vi "Positioncontrol_twomotor_pid.vi"() -> ()   [LabVIEW 2014]
uses:
  <vilib>/rvi/FXPMathLib/FxpSinAndCos/XNode/nifxpmath_SinAndCos.xnode
  <vilib>/eio/EIONode/EIONode.xnode
  <vilib>/rvi/FXPMathLib/FxpMul/XNode/nifxpmath_Multiplier.xnode
  <vilib>/rvi/FXPMathLib/FxpSinAndCos/simVIs/DllFxpSinAndCosTemp_sub.vi
  <vilib>/rvi/FXPMathLib/FxpSinAndCos/subVIs/nifxpmath_SinAndCos_SimConfig.ctl
  <vilib>/rvi/eio/common/nirviEmuTemplateMethod_errors.vi
  <vilib>/rvi/FXPMathLib/sim/FxpSim.dll
  <vilib>/rvi/DataTransferAndStorage/Container/XNode/niFpgaContainer.xnode
  <vilib>/rvi/FXPMathLib/FxpSub/XNode/nifxpmath_Sub.xnode
  <vilib>/rvi/FXPMathLib/FxpAdd/XNode/nifxpmath_Add.xnode
  <vilib>/rvi/Analysis/measure/butterworth/XNode/niFpgaButterworthFilter.xnode
  <vilib>/rvi/interface/RandomDataEmulation/nirviRandomDataFpgaReadWriteTemplate.vi
  <vilib>/rvi/interface/RandomDataEmulation/nirviRandomDataFpgaMultiElementTemplate.vi
panel:
  in  "Ramp_start":bool
  out "Dyr_slope":fxp<+/-,12,8>
  out "Dpr_slope":fxp<+/-,12,8>
  in  "Dyr_end":fxp<+/-,20,10>
  in  "Dyr_time":fxp<+/-,41,11>
  in  "Dpr_end":fxp<+/-,20,10>
  in  "Dpr_time":fxp<+/-,41,11>
  out "Dyr_ramp":fxp<+/-,12,7> format="%.18g"
  out "Dpr_ramp":fxp<+/-,12,7> format="%.18g"
  in  "Dyr_sin/cons":bool
  in  "Dpr_sin/cons":bool
  in  "Sin_magnitude":fxp<+/-,12,8>
  in  "Sin_offset":fxp<+/-,12,8>
  out "Dyr_sin":fxp<+/-,22,7> format="%.18g"
  out "Dpr_sin":fxp<+/-,22,7> format="%.18g"
  in  "Sin_period(sec)":fxp<+,10,8> format="%.21g"
  in  "Time_reset":bool
  in  "coe_ini":bool
  out "Dpt_i":fxp<+/-,25,11>
  out "Dyt_i":fxp<+/-,25,11>
  out "time now":fxp<+/-,41,11>
  in  "D_comp/tune_p":bool
  in  "D_comp/tune_y":bool
  in  "kp t":fxp<+,15,8>
  in  "kp c":fxp<+,15,8>
  in  "Kpp gain":fxp<+,27,10>=0.40625
  in  "Kpp slope gain":fxp<+,20,1>=0.40625
  in  "Kdp 2":fxp<+,27,10>
  in  "Kip 2":fxp<+,27,10>
  in  "I_comp/tune_p":bool
  out "Kpp":fxp<+,12,6>
  out "Kdp":fxp<+,34,10> format="%.25g"
  out "Kip":fxp<+,27,10> format="%.21g"
  in  "tolerance_Dp":fxp<+,12,2>=1.0
  in  "viscous_cons_p":fxp<+/-,20,10>
  in  "fcp":fxp<+/-,15,6>
  in  "fvp":fxp<+,20,12>
  in  "fv_coeff. p":fxp<+,13,1>
  in  "Dp_d_tol":fxp<+,20,12>
  in  "fstp":fxp<+/-,15,6>
  out "Dpr":fxp<+/-,22,7> format="%.18g"
  out "Friction comp_p":fxp<+/-,20,10>
  out "Fp_PID":fxp<+/-,20,10>
  out "Dp_tilde":fxp<+/-,33,9>
  out "xp_d":fxp<+/-,25,15>
  out "Dpt_d":fxp<+/-,25,15>
  out "Dp_d":fxp<+/-,25,15>
  out "vd_p_F":fxp<+/-,20,5>
  out "vq_p_F":fxp<+/-,20,5> format="%.57g"
  in  "Stop motor_p":bool
  out "va_p":fxp<+/-,20,5> format="%.21g"
  out "vb_p":fxp<+/-,20,5> format="%.21g"
  out "omega_p":fxp<+/-,20,9>
  in  "Encoder Reset_p":bool
  out "Encoder Position_p":i32
  out "rad(NrTheta)_p":fxp<+/-,33,18> format="%.21g"
  out "Dp(mm)":fxp<+/-,22,7>
  in  "viscous_cons_y":fxp<+/-,20,10>
  in  "I_comp/tune_y":bool
  in  "fsty":fxp<+/-,15,6>
  out "Dy_d":fxp<+/-,25,15>
  out "Dyr":fxp<+/-,22,7> format="%.18g"
  in  "Dy_d_tol":fxp<+,20,12>
  out "Dy_tilde":fxp<+/-,33,9>
  out "Dyt_d":fxp<+/-,25,15>
  in  "Kiy 2":fxp<+,27,10>
  in  "Kdy 2":fxp<+,27,10>
  in  "ky c":fxp<+,15,8>
  in  "ky t":fxp<+,15,8>
  out "Kiy":fxp<+,27,10> format="%.21g"
  in  "Kpy slope gain":fxp<+,20,1>=0.40625
  in  "Kpy gain":fxp<+,27,10>=0.40625
  in  "fv_coeff. y":fxp<+,13,1>
  out "Friction comp_y":fxp<+/-,20,10>
  in  "fcy":fxp<+/-,15,6>
  in  "fvy":fxp<+,20,12>
  out "xy_d":fxp<+/-,25,15>
  out "AI samp time (us)":u8
  out "x_p":fxp<+/-,30,6> format="%.40g"
  in  "Linear Sensor Reset_y":bool
  in  "kp":fxp<+,15,8>
  out "fp":fxp<+/-,20,10>
  in  "ky":fxp<+,15,8>
  out "fy":fxp<+/-,20,10>
  out "x_y":fxp<+/-,30,6>
  out "Kdy":fxp<+,34,10> format="%.25g"
  out "Kpy":fxp<+,12,6>
  out "Fy_PID":fxp<+/-,20,10>
  in  "tolerance_Dy":fxp<+,12,2>=1.0
  in  "Encoder Reset_y":bool
  out "Encoder Position_y":i32
  out "rad(NrTheta)_y":fxp<+/-,33,18> format="%.21g"
  out "Dy(mm)":fxp<+/-,22,7>
  out "omega_y":fxp<+/-,20,9>
  out "vq_y_F":fxp<+/-,20,5> format="%.57g"
  out "vd_y_F":fxp<+/-,20,5>
  in  "Stop motor_y":bool
  out "va_y":fxp<+/-,20,5> format="%.21g"
  out "vb_y":fxp<+/-,20,5> format="%.21g"
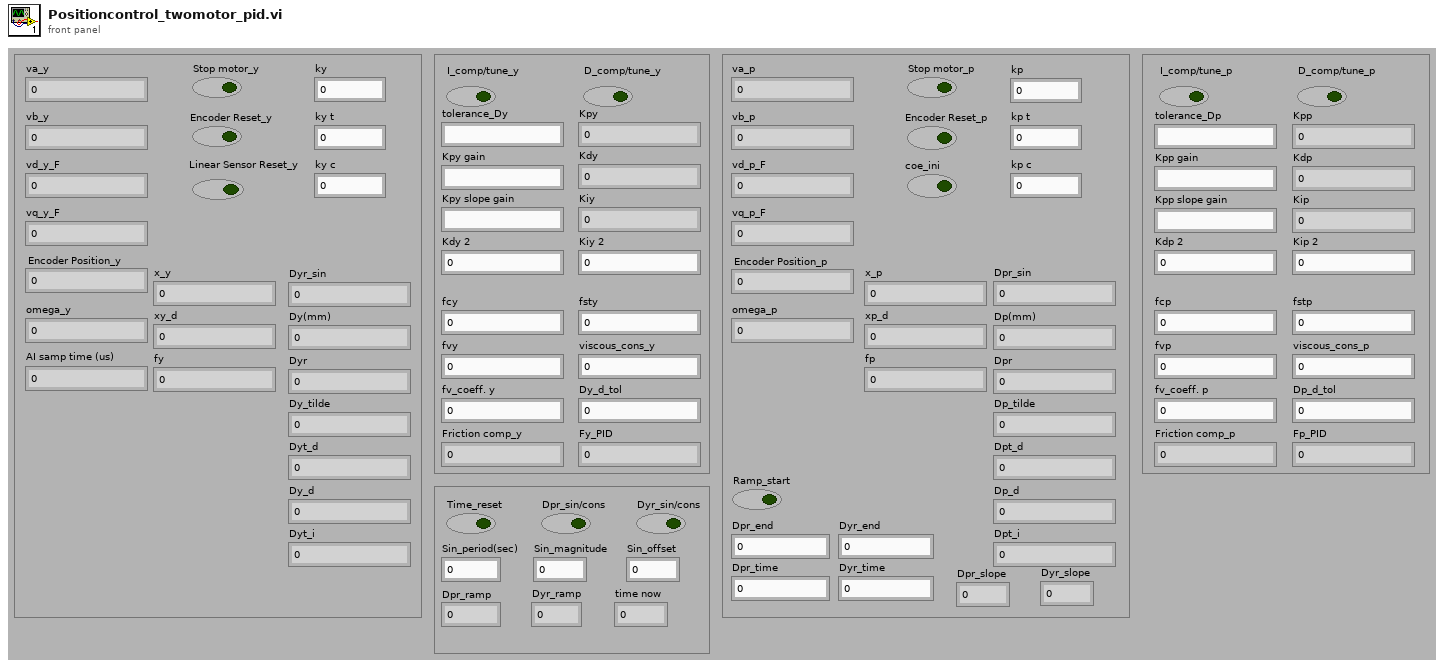
[diagram p1: front panel]
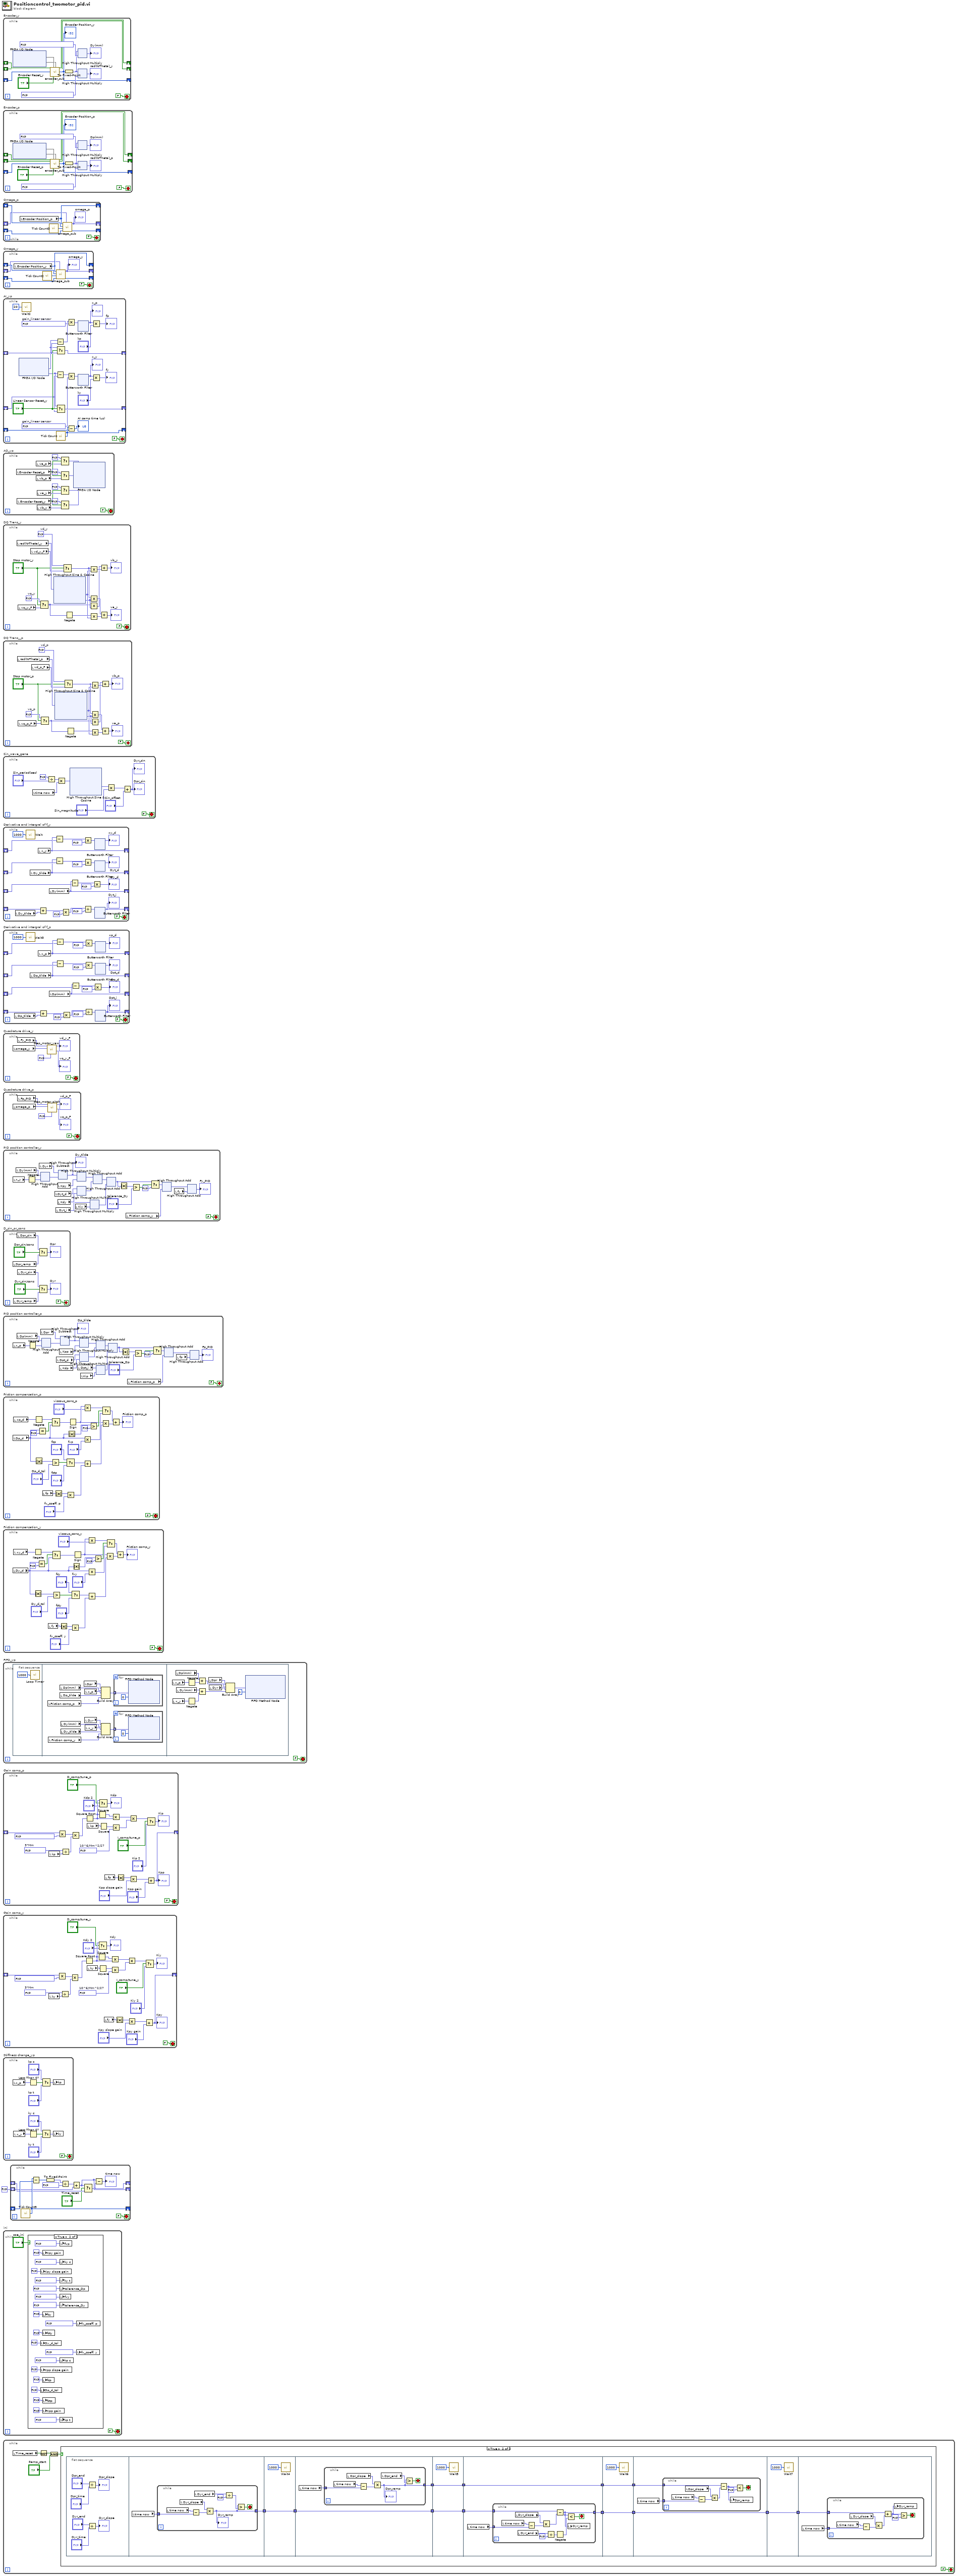
[diagram p0: block diagram]
diagram:
  n1 = while "Encoder_y" {
    shift-right: [w15] -> _
    shift-left: _ -> [w13]
    shift-right: [w14] -> _
    shift-left: _ -> [w12]
    shift-right: [w2] -> _
    shift-left: _ -> [w8]
    stop <- FALSE stop-if-true
    n2 = xnode "FPGA I/O Node"() -> ("Mod3/DIO2"=w11, "Mod3/DIO3"=w10)  [unwired: 2 in, 2 out]
    n3 = call "encoder_sub.vi"("A_pre"=w13, "B_pre"=w12, "Encoder Position_pre"=w8, "A input"=w11, "Encoder Position Reset"="Encoder Reset_y", "B input"=w10) -> ("A"=w15:bool, "B"=w14:bool, "Encoder Position (Counts)"=w2:i32)  [unwired: 19 in]
    "Encoder Position_y" <- w2
    n4 = To Fixed-Point(number=w2) -> (fixed-point=w5:fxp<+/-,18,18>)  [unwired: 1 in]
    n5 = xnode ("High Throughput Multiply")("x"=w5, "y"=fxp<+/-,15,-9> -0.0006049871444702148) -> ("x*y"=→"Dy(mm)":fxp<+/-,21,6>)
    n6 = xnode ("High Throughput Multiply")("x"=w5, "y"=fxp<+,24,0> 0.02499997615814209) -> ("x*y"=→"rad(NrTheta)_y":fxp<+/-,33,18>)
  }
  n7 = while "Encoder_p" {
    shift-right: [w30] -> _
    shift-left: _ -> [w28]
    shift-right: [w29] -> _
    shift-left: _ -> [w27]
    shift-right: [w17] -> _
    shift-left: _ -> [w23]
    stop <- FALSE stop-if-true
    n8 = xnode "FPGA I/O Node"() -> ("Mod3/DIO0"=w26, "Mod3/DIO1"=w25)  [unwired: 2 in, 2 out]
    n9 = call "encoder_sub.vi"("A_pre"=w28, "B_pre"=w27, "Encoder Position_pre"=w23, "A input"=w26, "Encoder Position Reset"="Encoder Reset_p", "B input"=w25) -> ("A"=w30:bool, "B"=w29:bool, "Encoder Position (Counts)"=w17:i32)  [unwired: 19 in]
    "Encoder Position_p" <- w17
    n10 = To Fixed-Point(number=w17) -> (fixed-point=w20:fxp<+/-,18,18>)  [unwired: 1 in]
    n11 = xnode ("High Throughput Multiply")("x"=w20, "y"=fxp<+/-,15,-9> -0.0006049871444702148) -> ("x*y"=→"Dp(mm)":fxp<+/-,21,6>)
    n12 = xnode ("High Throughput Multiply")("x"=w20, "y"=fxp<+,24,0> 0.02499997615814209) -> ("x*y"=→"rad(NrTheta)_p":fxp<+/-,33,18>)
  }
  n13 = while "Omega_p" {
    shift-right: [w39] -> _
    shift-left: _ -> [w38]
    shift-right: [w37] -> _
    shift-left: _ -> [w36]
    shift-right: [w34] -> _
    shift-left: _ -> [w35]
    stop <- FALSE stop-if-true
    n14 = local read "Encoder Position_p"() -> (w39:i32)
    n15 = call "Tick Count3"() -> ("Tick Count(Ticks)"=w32:u32)
    n16 = call "omega_sub.vi"("omega_pre"=w35, "ticks_m_pre"=w36, "ticks"=w32, "count_pre"=w38, "count"=w39) -> ("ticks_m"=w37:u32, "omega"=w34:fxp<+/-,20,9>)  [unwired: 4 in, 1 out]
    "omega_p" <- w34
  }
  n17 = while "Omega_y" {
    shift-right: [w47] -> _
    shift-left: _ -> [w46]
    shift-right: [w45] -> _
    shift-left: _ -> [w44]
    shift-right: [w42] -> _
    shift-left: _ -> [w43]
    stop <- FALSE stop-if-true
    n18 = local read "Encoder Position_y"() -> (w47:i32)
    n19 = call "Tick Count2"() -> ("Tick Count(Ticks)"=w40:u32)
    n20 = call "omega_sub.vi"("omega_pre"=w43, "ticks_m_pre"=w44, "ticks"=w40, "count_pre"=w46, "count"=w47) -> ("ticks_m"=w45:u32, "omega"=w42:fxp<+/-,20,9>)  [unwired: 4 in, 1 out]
    "omega_y" <- w42
  }
  n21 = while "AI_yp" {
    shift-right: [w70] -> _
    shift-left: _ -> [w71]
    shift-right: [w66] -> _
    shift-left: _ -> [w67]
    shift-right: [w61] -> _
    shift-left: _ -> [w60]
    stop <- FALSE stop-if-true
    w48 = fxp<+,25,5> 1.4694995880126953  # gain_linear sensor
    w57 = fxp<+,25,5> 1.5044002532958984  # gain_linear sensor
    n22 = xnode "FPGA I/O Node"() -> ("Mod1/AI0"=w63:fxp<+/-,20,5>, "Mod1/AI1"=w59:fxp<+/-,20,5>)  [unwired: 3 in, 3 out]
    n23 = call "Wait2"("Count(uSec)"=u8 20) -> ()  [unwired: 1 out]
    n24 = Subtract(x=w63, y=w67) -> (x-y=w54:fxp<+/-,21,6>)
    n25 = Subtract(x=w59, y=w60) -> (x-y=w58:fxp<+/-,21,6>)
    n26 = Select(t=w63, s="Linear Sensor Reset_y", f=w67) -> (s? t:f=w66:fxp<+/-,20,5>)
    n27 = Select(t=w59, s="Linear Sensor Reset_y", f=w60) -> (s? t:f=w61:fxp<+/-,20,5>)
    n28 = call "Tick Count"() -> ("Tick Count(uSec)"=w70:u8)
    n29 = Multiply(x=w54, y=w48) -> (x*y=w52:fxp<+/-,30,6>)
    n30 = Multiply(x=w58, y=w57) -> (x*y=w50:fxp<+/-,30,6>)
    n31 = Subtract(x=w70, y=w71) -> (x-y=→"AI samp time (us)":u8)
    n32 = xnode "Butterworth Filter"("input data"=w52) -> ("output data"=w51:fxp<+/-,30,6>)  [unwired: 2 in]
    "x_p" <- w51
    n33 = xnode "Butterworth Filter"("input data"=w50) -> ("output data"=w49:fxp<+/-,30,6>)  [unwired: 2 in]
    "x_y" <- w49
    n34 = Multiply(x=w51, y="kp") -> (x*y=→"fp":fxp<+/-,20,10>)
    n35 = Multiply(x=w49, y="ky") -> (x*y=→"fy":fxp<+/-,20,10>)
  }
  n36 = while "AO_yp" {
    stop <- FALSE stop-if-true
    n37 = local read "Encoder Reset_p"() -> (w101:bool)
    n38 = local read "Encoder Reset_y"() -> (w90:bool)
    n39 = local read "va_p"() -> (w100:fxp<+/-,20,5>)
    n40 = local read "vb_p"() -> (w99:fxp<+/-,20,5>)
    n41 = local read "va_y"() -> (w91:fxp<+/-,20,5>)
    n42 = local read "vb_y"() -> (w92:fxp<+/-,20,5>)
    n43 = Select(t=fxp<+/-,20,5> 5.0 ("Mod2/AO4"), s=w101, f=w100) -> (s? t:f=w96:fxp<+/-,20,5>)
    n44 = Select(t=fxp<+/-,20,5> 0.0 ("Mod2/AO4"), s=w101, f=w99) -> (s? t:f=w95:fxp<+/-,20,5>)
    n45 = Select(t=fxp<+/-,20,5> 5.0 ("Mod2/AO4"), s=w90, f=w91) -> (s? t:f=w89:fxp<+/-,20,5>)
    n46 = Select(t=fxp<+/-,20,5> 0.0 ("Mod2/AO4"), s=w90, f=w92) -> (s? t:f=w88:fxp<+/-,20,5>)
    n47 = xnode "FPGA I/O Node"("Mod2/AO0"=w96, "Mod2/AO1"=w95, "Mod2/AO2"=w89, "Mod2/AO3"=w88) -> ()  [unwired: 4 in, 4 out]
  }
  n48 = while "DQ Trans_y" {
    stop <- FALSE stop-if-true
    w108 = fxp<+/-,20,5> 0.0  # vq_y
    w106 = fxp<+/-,20,5> 0.0  # vd_y
    n49 = local read "rad(NrTheta)_y"() -> (w119:fxp<+/-,33,18>)
    n50 = local read "vq_y_F"() -> (w104:fxp<+/-,20,5>)
    n51 = local read "vd_y_F"() -> (w105:fxp<+/-,20,5>)
    n52 = Select(t=w108, s="Stop motor_y", f=w104) -> (s? t:f=w109:fxp<+/-,20,5>)
    n53 = xnode "High Throughput Sine & Cosine"("x (pi)"=w119) -> ("sin(x)"=w110:fxp<+/-,17,2>, "cos(x)"=w111:fxp<+/-,17,2>)
    n54 = Select(t=w106, s="Stop motor_y", f=w105) -> (s? t:f=w107:fxp<+/-,20,5>)
    n55 = Negate(x=w109) -> (-x=w118:fxp<+/-,21,6>)
    n56 = Multiply(x=w107, y=w110) -> (x*y=w114:fxp<+/-,20,5>)
    n57 = Multiply(x=w107, y=w111) -> (x*y=w117:fxp<+/-,20,5>)
    n58 = Multiply(x=w109, y=w111) -> (x*y=w113:fxp<+/-,20,5>)
    n59 = Multiply(x=w118, y=w110) -> (x*y=w116:fxp<+/-,20,5>)
    n60 = Add(x=w113, y=w114) -> (x+y=→"vb_y":fxp<+/-,20,5>)
    n61 = Add(x=w117, y=w116) -> (x+y=→"va_y":fxp<+/-,20,5>)
  }
  n62 = while "DQ Trans__p" {
    stop <- FALSE stop-if-true
    w158 = fxp<+/-,20,5> 0.0  # vq_p
    w156 = fxp<+/-,20,5> 0.0  # vd_p
    n63 = local read "rad(NrTheta)_p"() -> (w167:fxp<+/-,33,18>)
    n64 = local read "vq_p_F"() -> (w154:fxp<+/-,20,5>)
    n65 = local read "vd_p_F"() -> (w155:fxp<+/-,20,5>)
    n66 = Select(t=w158, s="Stop motor_p", f=w154) -> (s? t:f=w159:fxp<+/-,20,5>)
    n67 = xnode "High Throughput Sine & Cosine"("x (pi)"=w167) -> ("sin(x)"=w160:fxp<+/-,17,2>, "cos(x)"=w161:fxp<+/-,17,2>)
    n68 = Select(t=w156, s="Stop motor_p", f=w155) -> (s? t:f=w157:fxp<+/-,20,5>)
    n69 = Negate(x=w159) -> (-x=w166:fxp<+/-,21,6>)
    n70 = Multiply(x=w157, y=w160) -> (x*y=w163:fxp<+/-,20,5>)
    n71 = Multiply(x=w157, y=w161) -> (x*y=w165:fxp<+/-,20,5>)
    n72 = Multiply(x=w159, y=w161) -> (x*y=w162:fxp<+/-,20,5>)
    n73 = Multiply(x=w166, y=w160) -> (x*y=w164:fxp<+/-,20,5>)
    n74 = Add(x=w162, y=w163) -> (x+y=→"vb_p":fxp<+/-,20,5>)
    n75 = Add(x=w165, y=w164) -> (x+y=→"va_p":fxp<+/-,20,5>)
  }
  n76 = while "Sin_wave_gene" {
    stop <- FALSE stop-if-true
    n77 = local read "time now"() -> (w208:fxp<+/-,41,11>)
    n78 = Divide(x=fxp<+,10,8> 2.0, y="Sin_period(sec)") -> (x/y=w207:fxp<+/-,20,11>)
    n79 = Multiply(x=w207, y=w208) -> (x*y=w206:fxp<+/-,25,11>)
    n80 = xnode "High Throughput Sine & Cosine"("x (pi)"=w206) -> ("sin(x)"=w204:fxp<+/-,17,2>)  [unwired: 1 out]
    n81 = Multiply(x=w204, y="Sin_magnitude") -> (x*y=w202:fxp<+/-,20,8>)
    n82 = Add(x=w202, y="Sin_offset") -> (x+y=→"Dyr_sin" →"Dpr_sin":fxp<+/-,22,7>)
  }
  n83 = while "Derivative and intergral of f_y" {
    shift-right: [w261] -> _
    shift-left: _ -> [w260]
    shift-right: [w257] -> _
    shift-left: _ -> [w258]
    shift-right: [w250] -> _
    shift-left: _ -> [w249]
    shift-right: [w240] -> _
    shift-left: _ -> [w241]
    stop <- FALSE stop-if-true
    n84 = local read "Dy_tilde"() -> (w242:fxp<+/-,33,9>)
    n85 = call "Wait"("Count(uSec)"=u32 1000 ("Count(mSec)")) -> ()  [unwired: 1 out]
    n86 = local read "Dy_tilde"() -> (w257:fxp<+/-,33,9>)
    n87 = local read "x_y"() -> (w261:fxp<+/-,30,6>)
    n88 = Add(x=w241, y=w242) -> (x+y=w243:fxp<+/-,36,12>)
    n89 = local read "Dy(mm)"() -> (w250:fxp<+/-,22,7>)
    n90 = Subtract(x=w261, y=w260) -> (x-y=w263:fxp<+/-,31,7>)
    n91 = Subtract(x=w257, y=w258) -> (x-y=w254:fxp<+/-,34,10>)
    n92 = Multiply(x=w243, y=fxp<+/-,22,12> 0.5) -> (x*y=w245:fxp<+/-,25,15>)
    n93 = Subtract(x=w250, y=w249) -> (x-y=w252:fxp<+/-,23,8>)
    n94 = Multiply(x=w263, y=fxp<+,10,10> 1000.0) -> (x*y=w262:fxp<+/-,25,15>)
    n95 = Multiply(x=w254, y=fxp<+,10,10> 1000.0) -> (x*y=w256:fxp<+/-,25,15>)
    n96 = Divide(x=w245, y=fxp<+/-,25,15> 1000.0) -> (x/y=w247:fxp<+/-,25,11>)
    n97 = Multiply(x=w252, y=fxp<+,10,10> 1000.0) -> (x*y=→"Dy_d":fxp<+/-,25,15>)
    n98 = xnode "Butterworth Filter"("input data"=w262) -> ("output data"=→"xy_d":fxp<+/-,25,15>)  [unwired: 2 in]
    n99 = xnode "Butterworth Filter"("input data"=w256) -> ("output data"=→"Dyt_d":fxp<+/-,25,15>)  [unwired: 2 in]
    n100 = xnode "Butterworth Filter"("input data"=w247) -> ("output data"=w240:fxp<+/-,25,11>)  [unwired: 2 in]
    "Dyt_i" <- w240
  }
  n101 = while "Derivative and intergral of f_p" {
    shift-right: [w312] -> _
    shift-left: _ -> [w311]
    shift-right: [w308] -> _
    shift-left: _ -> [w309]
    shift-right: [w301] -> _
    shift-left: _ -> [w300]
    shift-right: [w291] -> _
    shift-left: _ -> [w292]
    stop <- FALSE stop-if-true
    n102 = local read "Dp_tilde"() -> (w298:fxp<+/-,33,9>)
    n103 = call "Wait3"("Count(uSec)"=u32 1000 ("Count(mSec)")) -> ()  [unwired: 1 out]
    n104 = local read "Dp_tilde"() -> (w308:fxp<+/-,33,9>)
    n105 = local read "x_p"() -> (w312:fxp<+/-,30,6>)
    n106 = Add(x=w292, y=w298) -> (x+y=w297:fxp<+/-,36,12>)
    n107 = local read "Dp(mm)"() -> (w301:fxp<+/-,22,7>)
    n108 = Subtract(x=w312, y=w311) -> (x-y=w314:fxp<+/-,31,7>)
    n109 = Subtract(x=w308, y=w309) -> (x-y=w305:fxp<+/-,34,10>)
    n110 = Multiply(x=w297, y=fxp<+/-,22,12> 0.5) -> (x*y=w295:fxp<+/-,25,15>)
    n111 = Subtract(x=w301, y=w300) -> (x-y=w303:fxp<+/-,23,8>)
    n112 = Multiply(x=w314, y=fxp<+,10,10> 1000.0) -> (x*y=w313:fxp<+/-,25,15>)
    n113 = Multiply(x=w305, y=fxp<+,10,10> 1000.0) -> (x*y=w307:fxp<+/-,25,15>)
    n114 = Divide(x=w295, y=fxp<+/-,25,15> 1000.0) -> (x/y=w293:fxp<+/-,25,11>)
    n115 = Multiply(x=w303, y=fxp<+,10,10> 1000.0) -> (x*y=→"Dp_d":fxp<+/-,25,15>)
    n116 = xnode "Butterworth Filter"("input data"=w313) -> ("output data"=→"xp_d":fxp<+/-,25,15>)  [unwired: 2 in]
    n117 = xnode "Butterworth Filter"("input data"=w307) -> ("output data"=→"Dpt_d":fxp<+/-,25,15>)  [unwired: 2 in]
    n118 = xnode "Butterworth Filter"("input data"=w293) -> ("output data"=w291:fxp<+/-,25,11>)  [unwired: 2 in]
    "Dpt_i" <- w291
  }
  n119 = while "Quadrature drive_y" {
    stop <- FALSE stop-if-true
    n120 = local read "omega_y"() -> (w345:fxp<+/-,20,9>)
    n121 = local read "Fy_PID"() -> (w346:fxp<+/-,20,10>)
    n122 = call "step_motor_yaw.vi"("F_Threshold"=fxp<+,12,12> 10.0, "omega_y"=w345, "F"=w346) -> ("vq_F"=→"vq_y_F":fxp<+/-,20,5>, "vd_F"=→"vd_y_F":fxp<+/-,20,5>)  [unwired: 7 in]
  }
  n123 = while "Quadrature drive_p" {
    stop <- FALSE stop-if-true
    n124 = local read "omega_p"() -> (w350:fxp<+/-,20,9>)
    n125 = local read "Fp_PID"() -> (w352:fxp<+/-,20,10>)
    n126 = call "step_motor_pitch.vi"("F_Threshold"=fxp<+,12,12> 10.0, "omega_p"=w350, "F"=w352) -> ("vq_F"=→"vq_p_F":fxp<+/-,20,5>, "vd_F"=→"vd_p_F":fxp<+/-,20,5>)  [unwired: 7 in]
  }
  n127 = while "PID position controller_y" {
    stop <- FALSE stop-if-true
    n128 = local read "x_y"() -> (w356:fxp<+/-,30,6>)
    n129 = local read "Dy(mm)"() -> (w355:fxp<+/-,22,7>)
    n130 = Negate(x=w356) -> (-x=w357:fxp<+/-,31,7>)
    n131 = local read "Dyr"() -> (w370:fxp<+/-,22,7>)
    n132 = xnode ("High Throughput Add")("x"=w355, "y"=w357) -> ("x+y"=w354:fxp<+/-,32,8>)
    n133 = local read "Dyt_d"() -> (w366:fxp<+/-,25,15>)
    n134 = local read "Dyt_i"() -> (w364:fxp<+/-,25,11>)
    n135 = local read "Kpy"() -> (w368:fxp<+,12,6>)
    n136 = local read "Kdy"() -> (w367:fxp<+,34,10>)
    n137 = xnode "High Throughput Subtract"("x"=w370, "y"=w354) -> ("x-y"=w369:fxp<+/-,33,9>)
    "Dy_tilde" <- w369
    n138 = local read "Kiy"() -> (w365:fxp<+,27,10>)
    n139 = xnode ("High Throughput Multiply")("x"=w369, "y"=w368) -> ("x*y"=w363:fxp<+/-,45,15>)
    n140 = xnode ("High Throughput Multiply")("x"=w366, "y"=w367) -> ("x*y"=w362:fxp<+/-,59,25>)
    n141 = xnode ("High Throughput Multiply")("x"=w364, "y"=w365) -> ("x*y"=w361:fxp<+/-,52,21>)
    n142 = xnode ("High Throughput Add")("x"=w363, "y"=w362) -> ("x+y"=w360:fxp<+/-,60,26>)
    n143 = xnode ("High Throughput Add")("x"=w360, "y"=w361) -> ("x+y"=w359:fxp<+/-,20,10>)
    n144 = Absolute Value(x=w359) -> (abs(x)=w377:fxp<+,20,10>)
    n145 = local read "Friction comp_y"() -> (w371:fxp<+/-,20,10>)
    n146 = Greater?(x=w377, y="tolerance_Dy") -> (0:w376:bool)
    n147 = Select(t=w359, s=w376, f=fxp<+/-,20,10> 0.0) -> (s? t:f=w373:fxp<+/-,20,10>)
    n148 = xnode ("High Throughput Add")("x"=w373, "y"=w371) -> ("x+y"=w372:fxp<+/-,20,10>)
    n149 = local read "fy"() -> (w374:fxp<+/-,20,10>)
    n150 = xnode ("High Throughput Add")("x"=w372, "y"=w374) -> ("x+y"=→"Fy_PID":fxp<+/-,20,10>)
  }
  n151 = while "D_sin_or_cons" {
    stop <- FALSE stop-if-true
    n152 = local read "Dpr_ramp"() -> (w381:fxp<+/-,12,7>)
    n153 = local read "Dyr_ramp"() -> (w380:fxp<+/-,12,7>)
    n154 = local read "Dpr_sin"() -> (w383:fxp<+/-,22,7>)
    n155 = local read "Dyr_sin"() -> (w382:fxp<+/-,22,7>)
    n156 = Select(t=w383, s="Dpr_sin/cons", f=w381) -> (s? t:f=→"Dpr":fxp<+/-,22,7>)
    n157 = Select(t=w382, s="Dyr_sin/cons", f=w380) -> (s? t:f=→"Dyr":fxp<+/-,22,7>)
  }
  n158 = while "PID position controller_p" {
    stop <- FALSE stop-if-true
    n159 = local read "x_p"() -> (w392:fxp<+/-,30,6>)
    n160 = local read "Dp(mm)"() -> (w390:fxp<+/-,22,7>)
    n161 = Negate(x=w392) -> (-x=w391:fxp<+/-,31,7>)
    n162 = local read "Dpr"() -> (w403:fxp<+/-,22,7>)
    n163 = xnode ("High Throughput Add")("x"=w390, "y"=w391) -> ("x+y"=w389:fxp<+/-,32,8>)
    n164 = local read "Dpt_d"() -> (w406:fxp<+/-,25,15>)
    n165 = local read "Kpp"() -> (w404:fxp<+,12,6>)
    n166 = local read "Kdp"() -> (w405:fxp<+,34,10>)
    n167 = xnode "High Throughput Subtract"("x"=w403, "y"=w389) -> ("x-y"=w399:fxp<+/-,33,9>)
    "Dp_tilde" <- w399
    n168 = local read "Dpt_i"() -> (w408:fxp<+/-,25,11>)
    n169 = xnode ("High Throughput Multiply")("x"=w399, "y"=w404) -> ("x*y"=w409:fxp<+/-,45,15>)
    n170 = xnode ("High Throughput Multiply")("x"=w406, "y"=w405) -> ("x*y"=w410:fxp<+/-,59,25>)
    n171 = local read "Kip"() -> (w407:fxp<+,27,10>)
    n172 = xnode ("High Throughput Add")("x"=w409, "y"=w410) -> ("x+y"=w412:fxp<+/-,60,26>)
    n173 = xnode ("High Throughput Multiply")("x"=w408, "y"=w407) -> ("x*y"=w411:fxp<+/-,52,21>)
    n174 = xnode ("High Throughput Add")("x"=w412, "y"=w411) -> ("x+y"=w413:fxp<+/-,20,10>)
    n175 = Absolute Value(x=w413) -> (abs(x)=w400:fxp<+,20,10>)
    n176 = local read "Friction comp_p"() -> (w396:fxp<+/-,20,10>)
    n177 = Greater?(x=w400, y="tolerance_Dp") -> (0:w401:bool)
    n178 = Select(t=w413, s=w401, f=fxp<+/-,20,10> 0.0) -> (s? t:f=w397:fxp<+/-,20,10>)
    n179 = xnode ("High Throughput Add")("x"=w397, "y"=w396) -> ("x+y"=w394:fxp<+/-,20,10>)
    n180 = local read "fp"() -> (w395:fxp<+/-,20,10>)
    n181 = xnode ("High Throughput Add")("x"=w394, "y"=w395) -> ("x+y"=→"Fp_PID":fxp<+/-,20,10>)
  }
  n182 = while "Friction compensation_p" {
    stop <- FALSE stop-if-true
    n183 = local read "Dp_d"() -> (w421:fxp<+/-,25,15>)
    n184 = local read "xp_d"() -> (w416:fxp<+/-,25,15>)
    n185 = Negate(x=w416) -> (-x=w415:fxp<+/-,26,16>)
    n186 = Absolute Value(x=w421) -> (abs(x)=w434:fxp<+,25,15>)
    n187 = Equal?(x=w421, y=fxp<+/-,25,15> 0.0) -> (x = y?=w422:bool)
    n188 = local read "fp"() -> (w439:fxp<+/-,20,10>)
    n189 = Greater?(x=w434, y="Dp_d_tol") -> (0:w433:bool)
    n190 = Select(t=w415, s=w422, f=w421) -> (s? t:f=w420:fxp<+/-,26,16>)
    n191 = Absolute Value(x=w439) -> (abs(x)=w440:fxp<+,20,10>)
    n192 = Select(t="fcp", s=w433, f="fstp") -> (s? t:f=w431:fxp<+/-,15,6>)
    n193 = Multiply(x=w440, y="fv_coeff. p") -> (x*y=w438:fxp<+/-,20,10>)
    n194 = Absolute Value(x=w421) -> (abs(x)=w428:fxp<+,25,15>)
    n195 = Sign(1:w420) -> (0:w419:fxp<+/-,2,2>)
    n196 = Multiply(x=w419, y="viscous_cons_p") -> (x*y=w424:fxp<+/-,20,10>)
    n197 = Multiply(x=w421, y="fvp") -> (x*y=w426:fxp<+/-,20,10>)
    n198 = Add(x=w431, y=w438) -> (x+y=w437:fxp<+/-,20,10>)
    n199 = Greater?(x=w428, y=fxp<+/-,25,15> 25.0) -> (0:w427:bool)
    n200 = Multiply(x=w419, y=w437) -> (x*y=w436:fxp<+/-,20,10>)
    n201 = Select(t=w424, s=w427, f=w426) -> (s? t:f=w425:fxp<+/-,20,10>)
    n202 = Add(x=w425, y=w436) -> (x+y=→"Friction comp_p":fxp<+/-,20,10>)
  }
  n203 = while "Friction compensation_y" {
    stop <- FALSE stop-if-true
    n204 = local read "Dy_d"() -> (w448:fxp<+/-,25,15>)
    n205 = local read "xy_d"() -> (w445:fxp<+/-,25,15>)
    n206 = Negate(x=w445) -> (-x=w444:fxp<+/-,26,16>)
    n207 = Absolute Value(x=w448) -> (abs(x)=w462:fxp<+,25,15>)
    n208 = Equal?(x=w448, y=fxp<+/-,25,15> 0.0) -> (x = y?=w449:bool)
    n209 = local read "fy"() -> (w468:fxp<+/-,20,10>)
    n210 = Select(t=w444, s=w449, f=w448) -> (s? t:f=w447:fxp<+/-,26,16>)
    n211 = Greater?(x=w462, y="Dy_d_tol") -> (0:w461:bool)
    n212 = Absolute Value(x=w468) -> (abs(x)=w469:fxp<+,20,10>)
    n213 = Multiply(x=w469, y="fv_coeff. y") -> (x*y=w466:fxp<+/-,20,10>)
    n214 = Select(t="fcy", s=w461, f="fsty") -> (s? t:f=w459:fxp<+/-,15,6>)
    n215 = Absolute Value(x=w448) -> (abs(x)=w456:fxp<+,25,15>)
    n216 = Sign(1:w447) -> (0:w446:fxp<+/-,2,2>)
    n217 = Multiply(x=w446, y="viscous_cons_y") -> (x*y=w451:fxp<+/-,20,10>)
    n218 = Multiply(x=w448, y="fvy") -> (x*y=w454:fxp<+/-,20,10>)
    n219 = Add(x=w459, y=w466) -> (x+y=w465:fxp<+/-,20,10>)
    n220 = Greater?(x=w456, y=fxp<+/-,25,15> 25.0) -> (0:w455:bool)
    n221 = Multiply(x=w446, y=w465) -> (x*y=w464:fxp<+/-,20,10>)
    n222 = Select(t=w451, s=w455, f=w454) -> (s? t:f=w453:fxp<+/-,20,10>)
    n223 = Add(x=w453, y=w464) -> (x+y=→"Friction comp_y":fxp<+/-,20,10>)
  }
  n224 = while "FIFO_yp" {
    stop <- FALSE stop-if-true
    n225 = flat-sequence {
      frame #0 {
        n226 = call "Loop Timer"("Count(uSec)"=u32 1000 ("Loop Period (usec)")) -> ()  [unwired: 1 out]
      }
      frame #1 {
        n227 = local read "Friction comp_p"() -> (w476:fxp<+/-,20,10>)
        n228 = local read "Friction comp_y"() -> (w485:fxp<+/-,20,10>)
        n229 = local read "Dp(mm)"() -> (w479:fxp<+/-,22,7>)
        n230 = local read "Dp_tilde"() -> (w477:fxp<+/-,33,9>)
        n231 = local read "Dy(mm)"() -> (w482:fxp<+/-,22,7>)
        n232 = local read "Dy_tilde"() -> (w484:fxp<+/-,33,9>)
        n233 = local read "Dpr"() -> (w480:fxp<+/-,22,7>)
        n234 = local read "x_p"() -> (w478:fxp<+/-,30,6>)
        n235 = local read "Dyr"() -> (w481:fxp<+/-,22,7>)
        n236 = local read "x_y"() -> (w483:fxp<+/-,30,6>)
        n237 = Build Array(w480, w479, w478, w477, w476) -> (w475:fxp<+/-,34,10>[])
        n238 = Build Array(w481, w482, w483, w484, w485) -> (w486:fxp<+/-,34,10>[])
        n239 = for {
          tunnel: w475 -> [w487] mode=indexing
          n240 = xnode ("FIFO Method Node")("Element"=w487, "Timeout"=0) -> ()  [unwired: 1 in, 2 out]
        }
        n241 = for {
          tunnel: w486 -> [w489] mode=indexing
          n242 = xnode ("FIFO Method Node")("Element"=w489, "Timeout"=0) -> ()  [unwired: 1 in, 2 out]
        }
      }
      frame #2 {
        n243 = local read "x_p"() -> (w502:fxp<+/-,30,6>)
        n244 = local read "x_y"() -> (w493:fxp<+/-,30,6>)
        n245 = local read "Dp(mm)"() -> (w500:fxp<+/-,22,7>)
        n246 = local read "Dy(mm)"() -> (w495:fxp<+/-,22,7>)
        n247 = Negate(x=w502) -> (-x=w501:fxp<+/-,31,7>)
        n248 = Negate(x=w493) -> (-x=w494:fxp<+/-,31,7>)
        n249 = Add(x=w500, y=w501) -> (x+y=w498:fxp<+/-,32,8>)
        n250 = Add(x=w495, y=w494) -> (x+y=w492:fxp<+/-,32,8>)
        n251 = local read "Dpr"() -> (w499:fxp<+/-,22,7>)
        n252 = local read "Dyr"() -> (w491:fxp<+/-,22,7>)
        n253 = Build Array(w499, w498, w491, w492) -> (w497:fxp<+/-,32,8>[])
        n254 = xnode ("FIFO Method Node")("Element"=w497, "Timeout"=0) -> ()  [unwired: 1 in, 2 out]
      }
    }
  }
  n255 = while "Gain comp_p" {
    shift-right: [w507] -> _
    shift-left: _ -> [w526]
    stop <- FALSE stop-if-true
    w514 = fxp<+,14,7> 111.8125  # 10^6/Mm^2/27
    w529 = fxp<+,14,7> 54.6015625  # 3*Mm
    n256 = local read "kp"() -> (w528:fxp<+,15,8>)
    n257 = Multiply(x=w526, y=fxp<+,12,-6> 0.00099945068359375) -> (x*y=w525:fxp<+,24,0>)
    n258 = Divide(x=w529, y=w528) -> (x/y=w524:fxp<+,23,7>)
    n259 = Multiply(x=w525, y=w524) -> (x*y=w523:fxp<+,32,0>)
    n260 = Square Root(x=w523) -> (sqrt(x)=w510:fxp<+,26,2>)
    n261 = local read "kp"() -> (w515:fxp<+,15,8>)
    n262 = Square(x=w510) -> (x^2=w517:fxp<+,27,3>)
    n263 = Select(t=w510, s="D_comp/tune_p", f="Kdp 2") -> (s? t:f=→"Kdp":fxp<+,34,10>)
    n264 = Square(x=w515) -> (x^2=w513:fxp<+,30,16>)
    n265 = local read "fp"() -> (w520:fxp<+/-,20,10>)
    n266 = Multiply(x=w517, y=w510) -> (x*y=w516:fxp<+,27,3>)
    n267 = Multiply(x=w513, y=w514) -> (x*y=w512:fxp<+,44,20>)
    n268 = Absolute Value(x=w520) -> (abs(x)=w521:fxp<+,20,10>)
    n269 = Multiply(x=w516, y=w512) -> (x*y=w509:fxp<+,27,10>)
    n270 = Multiply(x=w521, y="Kpp slope gain") -> (x*y=w519:fxp<+,12,4>)
    n271 = Add(x=w519, y="Kpp gain") -> (x+y=w507:fxp<+,12,6>)
    "Kpp" <- w507
    n272 = Select(t=w509, s="I_comp/tune_p", f="Kip 2") -> (s? t:f=→"Kip":fxp<+,27,10>)
  }
  n273 = while "Gain comp_y" {
    shift-right: [w545] -> _
    shift-left: _ -> [w554]
    stop <- FALSE stop-if-true
    w541 = fxp<+,14,7> 111.8125  # 10^6/Mm^2/27
    w557 = fxp<+,14,7> 54.6015625  # 3*Mm
    n274 = local read "ky"() -> (w556:fxp<+,15,8>)
    n275 = Multiply(x=w554, y=fxp<+,12,-6> 0.00099945068359375) -> (x*y=w553:fxp<+,24,0>)
    n276 = Divide(x=w557, y=w556) -> (x/y=w552:fxp<+,23,7>)
    n277 = Multiply(x=w553, y=w552) -> (x*y=w551:fxp<+,32,0>)
    n278 = Square Root(x=w551) -> (sqrt(x)=w536:fxp<+,26,2>)
    n279 = local read "ky"() -> (w542:fxp<+,15,8>)
    n280 = Square(x=w536) -> (x^2=w544:fxp<+,27,3>)
    n281 = Select(t=w536, s="D_comp/tune_y", f="Kdy 2") -> (s? t:f=→"Kdy":fxp<+,34,10>)
    n282 = Square(x=w542) -> (x^2=w540:fxp<+,30,16>)
    n283 = local read "fy"() -> (w548:fxp<+/-,20,10>)
    n284 = Multiply(x=w544, y=w536) -> (x*y=w543:fxp<+,27,3>)
    n285 = Multiply(x=w540, y=w541) -> (x*y=w539:fxp<+,44,20>)
    n286 = Absolute Value(x=w548) -> (abs(x)=w549:fxp<+,20,10>)
    n287 = Multiply(x=w543, y=w539) -> (x*y=w534:fxp<+,27,10>)
    n288 = Multiply(x=w549, y="Kpy slope gain") -> (x*y=w547:fxp<+,12,4>)
    n289 = Add(x=w547, y="Kpy gain") -> (x+y=w545:fxp<+,12,6>)
    "Kpy" <- w545
    n290 = Select(t=w534, s="I_comp/tune_y", f="Kiy 2") -> (s? t:f=→"Kiy":fxp<+,27,10>)
  }
  n291 = while "Stiffness change_yp" {
    stop <- FALSE stop-if-true
    n292 = local read "x_p"() -> (w559:fxp<+/-,30,6>)
    n293 = local read "x_y"() -> (w569:fxp<+/-,30,6>)
    n294 = Less Than 0?(x=w559) -> (x < 0?=w560:bool)
    n295 = Less Than 0?(x=w569) -> (x < 0?=w568:bool)
    n296 = Select(t="kp c", s=w560, f="kp t") -> (s? t:f=w561:fxp<+,15,8>)
    n297 = Select(t="ky c", s=w568, f="ky t") -> (s? t:f=w567:fxp<+,15,8>)
    n298 = local write "kp"(w561) -> ()
    n299 = local write "ky"(w567) -> ()
  }
  n300 = while "ini" {
    stop <- FALSE stop-if-true
    n301 = case shown="True" "coe_ini" {
      frame False {
      }
      frame True {
        n302 = local write "Kpy slope gain"(fxp<+,20,1> 0.0 ("Kpy slope gain")) -> ()
        n303 = local write "Dy_d_tol"(fxp<+,20,12> 3.0 ("Dy_d_tol")) -> ()
        n304 = local write "Kpp slope gain"(fxp<+,20,1> 0.0 ("Kpp slope gain")) -> ()
        n305 = local write "Dp_d_tol"(fxp<+,20,12> 3.0 ("Dp_d_tol")) -> ()
        n306 = local write "Kpy gain"(fxp<+,27,10> 10.0 ("Kpy gain")) -> ()
        n307 = local write "fcy"(fxp<+/-,15,6> 18.0 ("fcy")) -> ()
        n308 = local write "fsty"(fxp<+/-,15,6> 18.0 ("fsty")) -> ()
        n309 = local write "fcp"(fxp<+/-,15,6> 14.0 ("fcp")) -> ()
        n310 = local write "fstp"(fxp<+/-,15,6> 16.0 ("fstp")) -> ()
        n311 = local write "Kpp gain"(fxp<+,27,10> 10.0 ("Kpp gain")) -> ()
        n312 = local write "fvp"(fxp<+,20,12> 0.19921875 ("fvp")) -> ()
        n313 = local write "ky c"(fxp<+,15,8> 34.0234375 ("kp c")) -> ()
        n314 = local write "ky t"(fxp<+,15,8> 33.3359375 ("ky")) -> ()
        n315 = local write "tolerance_Dp"(fxp<+,12,2> 0.099609375 ("tolerance_p")) -> ()
        n316 = local write "fvy"(fxp<+,20,12> 0.19921875 ("fvy")) -> ()
        n317 = local write "tolerance_Dy"(fxp<+,12,2> 0.099609375 ("tolerance_y")) -> ()
        n318 = local write "kp c"(fxp<+,15,8> 36.2421875 ("kp c")) -> ()
        n319 = local write "kp t"(fxp<+,15,8> 31.8046875 ("kp t")) -> ()
        n320 = local write "fv_coeff. p"(fxp<+,13,1> 0.14990234375 ("fv_coeff. p")) -> ()
        n321 = local write "fv_coeff. y"(fxp<+,13,1> 0.14990234375 ("fv_coeff. y")) -> ()
      }
    }
  }
  n322 = while {
    stop <- FALSE stop-if-true
    n323 = local read "Time_reset"() -> (w595:bool)
    n324 = Not(x=w595) -> (.not. x?=w593:bool)
    n325 = And(x=w593, y="Ramp_start") -> (x .and. y?=w592:bool)
    n326 = case shown="True" w592 {
      frame False {
      }
      frame True {
        n327 = flat-sequence {
          tunnel: [w616] -> w608
          tunnel: w608 -> [w626]
          tunnel: [w626] -> w607
          tunnel: [w630] -> w606
          tunnel: w607 -> [w630]
          tunnel: [w629] -> w605
          tunnel: [w639] -> w604
          tunnel: w606 -> [w639]
          tunnel: [w638] -> w603
          tunnel: w605 -> [w638]
          tunnel: w604 -> [w644]
          tunnel: [w643] -> w602
          tunnel: w603 -> [w643]
          tunnel: [w642] -> w601
          tunnel: [w658] -> w600
          tunnel: w602 -> [w658]
          tunnel: w601 -> [w657]
          tunnel: [w657] -> w599
          tunnel: w600 -> [w662]
          tunnel: w599 -> [w661]
          tunnel: [w661] -> w598
          tunnel: w598 -> [w673]
          tunnel: [w673] -> w597
          tunnel: w597 -> [w675]
          frame #0 {
            n328 = Divide(x="Dpr_end", y="Dpr_time") -> (x/y=→"Dpr_slope":fxp<+/-,12,8>)
            n329 = Divide(x="Dyr_end", y="Dyr_time") -> (x/y=→"Dyr_slope":fxp<+/-,12,8>)
          }
          frame #1 {
            n330 = local read "time now"() -> (w615:fxp<+/-,41,11>)
            n331 = while {
              tunnel: [w621] -> w616
              tunnel: w615 -> [w618]
              stop <- w622 stop-if-true
              n332 = local read "time now"() -> (w619:fxp<+/-,41,11>)
              n333 = local read "Dyr_slope"() -> (w620:fxp<+/-,12,8>)
              n334 = Subtract(x=w619, y=w618) -> (x-y=w617:fxp<+/-,42,12>)
              n335 = local read "Dyr_end"() -> (w625:fxp<+/-,20,10>)
              n336 = Multiply(x=w620, y=w617) -> (x*y=w621:fxp<+/-,12,7>)
              "Dyr_ramp" <- w621
              n337 = Divide(x=w625, y=fxp<+/-,20,10> 2.0) -> (x/y=w623:fxp<+/-,41,21>)
              n338 = Greater?(x=w621, y=w623) -> (0:w622:bool)
            }
          }
          frame #2 {
            n339 = call "Wait4"("Count(mSec)"=u32 1000) -> ()  [unwired: 1 out]
          }
          frame #3 {
            n340 = local read "time now"() -> (w628:fxp<+/-,41,11>)
            n341 = while {
              tunnel: [w636] -> w629
              tunnel: w628 -> [w633]
              stop <- w637 stop-if-true
              n342 = local read "time now"() -> (w632:fxp<+/-,41,11>)
              n343 = local read "Dpr_slope"() -> (w634:fxp<+/-,12,8>)
              n344 = Subtract(x=w632, y=w633) -> (x-y=w631:fxp<+/-,42,12>)
              n345 = Multiply(x=w634, y=w631) -> (x*y=w636:fxp<+/-,12,7>)
              "Dpr_ramp" <- w636
              n346 = local read "Dpr_end"() -> (w635:fxp<+/-,20,10>)
              n347 = Greater?(x=w636, y=w635) -> (0:w637:bool)
            }
          }
          frame #4 {
            n348 = call "Wait5"("Count(mSec)"=u32 1000) -> ()  [unwired: 1 out]
          }
          frame #5 {
            n349 = local read "time now"() -> (w641:fxp<+/-,41,11>)
            n350 = while {
              tunnel: w644 -> [w651]
              tunnel: [w648] -> w642
              tunnel: w641 -> [w646]
              stop <- w652 stop-if-true
              n351 = local read "time now"() -> (w647:fxp<+/-,41,11>)
              n352 = local read "Dyr_slope"() -> (w650:fxp<+/-,12,8>)
              n353 = local read "Dyr_end"() -> (w655:fxp<+/-,20,10>)
              n354 = Subtract(x=w647, y=w646) -> (x-y=w645:fxp<+/-,42,12>)
              n355 = Multiply(x=w650, y=w645) -> (x*y=w649:fxp<+/-,12,7>)
              n356 = Divide(x=w655, y=fxp<+/-,20,10> 2.0) -> (x/y=w654:fxp<+/-,41,21>)
              n357 = Subtract(x=w651, y=w649) -> (x-y=w648:fxp<+/-,12,7>)
              n358 = Negate(x=w654) -> (-x=w653:fxp<+/-,41,21>)
              n359 = Less?(x=w648, y=w653) -> (x < y?=w652:bool)
              n360 = local write "Dyr_ramp"(w648) -> ()
            }
          }
          frame #6 {
            n361 = call "Wait6"("Count(mSec)"=u32 1000) -> ()  [unwired: 1 out]
          }
          frame #7 {
            n362 = local read "time now"() -> (w660:fxp<+/-,41,11>)
            n363 = while {
              tunnel: w662 -> [w667]
              tunnel: w660 -> [w664]
              stop <- w671 stop-if-true
              n364 = local read "time now"() -> (w665:fxp<+/-,41,11>)
              n365 = local read "Dpr_slope"() -> (w670:fxp<+/-,12,8>)
              n366 = Subtract(x=w665, y=w664) -> (x-y=w663:fxp<+/-,42,12>)
              n367 = Multiply(x=w670, y=w663) -> (x*y=w669:fxp<+/-,12,7>)
              n368 = Subtract(x=w667, y=w669) -> (x-y=w668:fxp<+/-,12,7>)
              n369 = local write "Dpr_ramp"(w668) -> ()
              n370 = Less?(x=w668, y=fxp<+/-,12,7> 0.0) -> (x < y?=w671:bool)
            }
          }
          frame #8 {
            n371 = call "Wait7"("Count(mSec)"=u32 1000) -> ()  [unwired: 1 out]
          }
          frame #9 {
            n372 = local read "time now"() -> (w674:fxp<+/-,41,11>)
            n373 = while {
              tunnel: w675 -> [w682]
              tunnel: w674 -> [w678]
              stop <- w679 stop-if-true
              n374 = local read "time now"() -> (w677:fxp<+/-,41,11>)
              n375 = local read "Dyr_slope"() -> (w684:fxp<+/-,12,8>)
              n376 = Subtract(x=w677, y=w678) -> (x-y=w676:fxp<+/-,42,12>)
              n377 = Multiply(x=w684, y=w676) -> (x*y=w683:fxp<+/-,12,7>)
              n378 = Add(x=w682, y=w683) -> (x+y=w680:fxp<+/-,12,7>)
              n379 = local write "Dyr_ramp"(w680) -> ()
              n380 = Greater?(x=w680, y=fxp<+/-,12,7> 0.0) -> (0:w679:bool)
            }
          }
        }
      }
    }
  }
  n381 = while {
    shift-right: [w696] -> _
    shift-left: _ -> [w697]
    shift-right: [w689] -> _
    shift-left: fxp<+,36,6> 0.0 -> [w695]
    shift-right: [w687] -> _
    shift-left: _ -> [w688]
    stop <- FALSE stop-if-true
    n382 = call "Tick Count5"() -> ("Tick Count(uSec)"=w696:u8)
    n383 = Subtract(x=w696, y=w697) -> (x-y=w693:u8)
    n384 = To Fixed-Point(number=w693) -> (fixed-point=w692:fxp<+,8,8>)  [unwired: 1 in]
    n385 = Divide(x=w692, y=fxp<+,14,20> 1000000.0) -> (x/y=w691:fxp<+,15,-15>)
    n386 = Add(x=w691, y=w695) -> (x+y=w689:fxp<+,40,10>)
    n387 = Select(t=w689, s="Time_reset", f=w688) -> (s? t:f=w687:fxp<+,40,10>)
    n388 = Subtract(x=w689, y=w687) -> (x-y=→"time now":fxp<+/-,41,11>)
  }
